vi "Pre Launch Init.vi"(11 "Tcp in":refnum<class "Tcp.lvclass">) -> (0 "error out":errorcluster, 3 "Tcp out":refnum<class "Tcp.lvclass">)   [LabVIEW 2022 SP3, in "Tcp.lvlib" / "Tcp.lvclass"]
doc: "(<B>Filename</B>: Actor Framework.lvlib:Actor.lvclass:Pre Launch Init.vi)\n\nDefines behavior that occurs after the Launch Actor method is invoked but before the actor's Actor Core method begins running.\n\nThe Pre Launch Init method is guaranteed to finish before the Launch Actor method returns to its caller and before the actor itself receives any messages. Any references that the Pre Launch Init method obtains are guaranteed to have the same lifetime as the actor itself. Any errors that the Pre Launch Init method returns will abort the launch.\n\nBy default, this method does nothing. A descendant class may override it to define behavior."
uses:
  Tcp.lvclass
  C:/Users/jakub/repos/gh/sw4sys/lv-cli-framework/LoggingActor/Source/LoggingActor/LoggingActor/LoggingActor.lvclass
  C:/Program Files (x86)/National Instruments/LabVIEW 2022/vi.lib/ActorFramework/Actor/Actor.lvclass
  LoggingActor/Source/LoggingActor/LoggingActor/LoggingActor.lvclass/LoggingActor.ctl
  TcpSocket/Source/TcpSocket/TcpSocket/TcpSocket.lvclass/TcpSocket.ctl
  Tcp.lvclass/Tcp.ctl
  <vilib>/ActorFramework/Actor/Actor.lvclass/Actor.ctl
  <vilib>/ActorFramework/Message Enqueuer/Message Enqueuer.lvclass/Message Enqueuer.ctl
  TcpSocket/Source/TcpSocket/TcpSocket/Read Address.vi
  TcpSocket/Source/TcpSocket/TcpSocket/Read Port.vi
  LoggingActor/Source/LoggingActor/LoggingActor/Read Logger.vi
  <vilib>/ActorFramework/Message Enqueuer/Init from Existing Queue.vi
  <vilib>/ActorFramework/Message Enqueuer/Enqueue.vi
  TcpSocket/Source/TcpSocket/TcpServer/TcpServer.lvclass
  C:/Users/jakub/repos/gh/sw4sys/lv-cli-framework/TcpSocket/Source/TcpSocket/TcpSocket/TcpSocket.lvclass
  Tcp Messages/WaitForConnection Msg/WaitForConnection Msg.lvclass
  C:/Program Files (x86)/National Instruments/LabVIEW 2022/vi.lib/ActorFramework/Message/Message.lvclass
  <vilib>/ActorFramework/Message Priority Queue/Priority Enqueue.vi
  LoggingActor/Source/LoggingActor/LoggingActor/LoggingActor.lvclass
  Logger/Source/Logger/Logger.lvclass
  <vilib>/ActorFramework/Message Enqueuer/Message Enqueuer.lvclass
  <vilib>/ActorFramework/Actor/Actor.lvclass
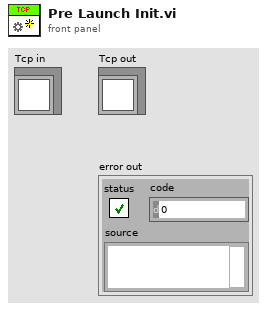
[diagram p1: front panel]
types:
  T1 = enum16{"Standard", "Buffered", "CRLF", "Immediate"}
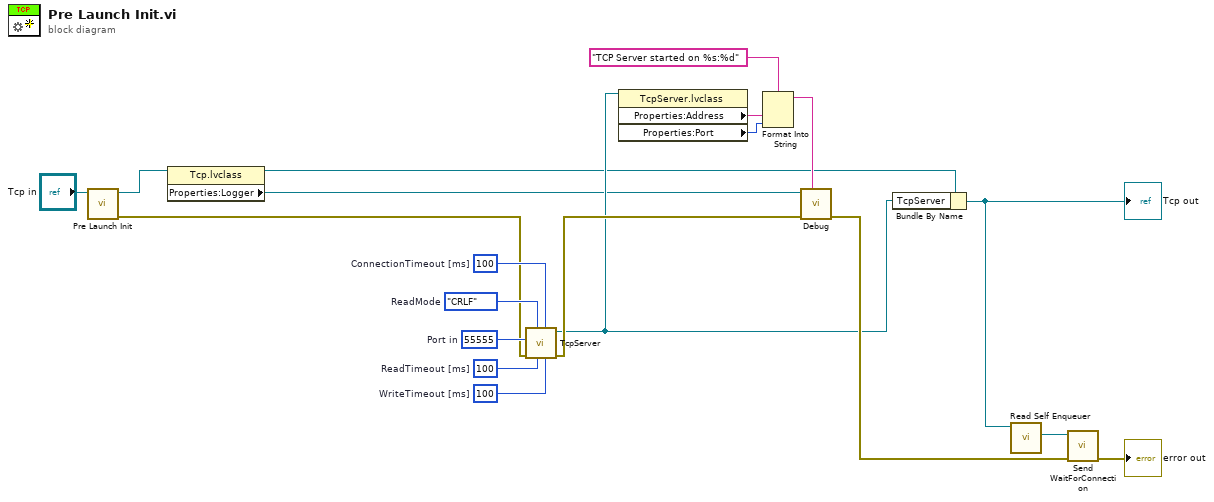
[diagram p0: block diagram]
diagram:
  w17 = 100  # ConnectionTimeout [ms]
  w18 = 100  # WriteTimeout [ms]
  w19 = 100  # ReadTimeout [ms]
  w20 = T1."CRLF"  # ReadMode
  w9 = u16 55555  # Port in
  n1 = call-parent "Pre Launch Init.vi"("LoggingActor in"="Tcp in") -> ("error out"=w4:errorcluster, "LoggingActor out"=w2:refnum<class "Tcp.lvclass">)  [unwired: 9 in]
  n2 = property class="Tcp.lvclass"(reference=w2) -> (reference out=w1:refnum<class "Tcp.lvclass">, "Properties:Logger"=w3:refnum<class "Logger.lvclass">)  [unwired: 1 in, 1 out]
  n3 = call "TcpServer.vi"("WriteTimeout [ms] (5000)"=w18, "ConnectionTimeout [ms] (5000)"=w17, "ReadTimeout [ms] (5000)"=w19, "ReadMode (Standard)"=w20, "error in (no error)"=w4, "Port in (0)"=w9) -> ("error out"=w12:errorcluster, "TcpServer"=w8:refnum<class "TcpServer.lvclass">)  [unwired: 3 in, 1 out]
  n4 = property class="TcpServer.lvclass"(reference=w8) -> ("Properties:Address"=w7:string, "Properties:Port"=w6:u16)  [unwired: 1 in, 2 out]
  n5 = Format Into String(format string="TCP Server started on %s:%d", w7, w6) -> (resulting string=w5:string)  [unwired: 2 in, 1 out]
  n6 = call-dynamic "Debug.vi"("Message"=w5, "error in (no error)"=w12, "Logger in"=w3) -> ("error out"=w11:errorcluster)  [unwired: 7 in, 1 out]
  n7 = Bundle By Name(cluster=w1, "TcpServer"=w8) -> (w16:refnum<class "Tcp.lvclass">)
  "Tcp out" <- w16
  n8 = call <vilib>:"Read Self Enqueuer.vi"("Actor"=w16) -> ("Self Enqueuer"=w15:refnum<class "Message Enqueuer.lvclass">)  [unwired: 10 in]
  n9 = call "Send WaitForConnection.vi"("error in (no error)"=w11, "Message Enqueuer"=w15) -> ("error out"=→"error out":errorcluster)  [unwired: 8 in, 1 out]
